vi "Error Cluster to Array.vi"(10 "error in (no error)":errorcluster) -> (2 "Error Array":string[](array[string]))   [LabVIEW 2019, in "Logger.Error.lvlib" / "Logger.Error.lvclass"]
uses:
  Logger.Error.lvclass
  <vilib>/Utility/error.llb/DialogType.ctl
  <userlib>/_OpenG.lib/string/string.llb/Trim Whitespace (String)__ogtk.vi
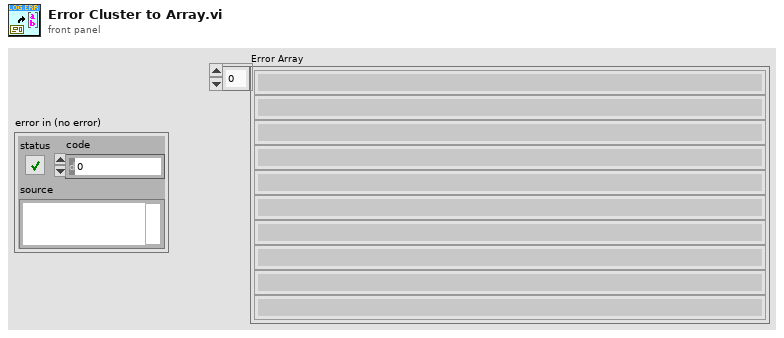
[diagram p1: front panel]
types:
  T1 = cluster{"Date":string, "Time":string, "Type":string, "Name":string, "Code":string, "Message":string, "Possible reason(s)":string, "Call Chain":string, "Calling Class":string}
  T2 = typedef "DialogType.ctl" = u16
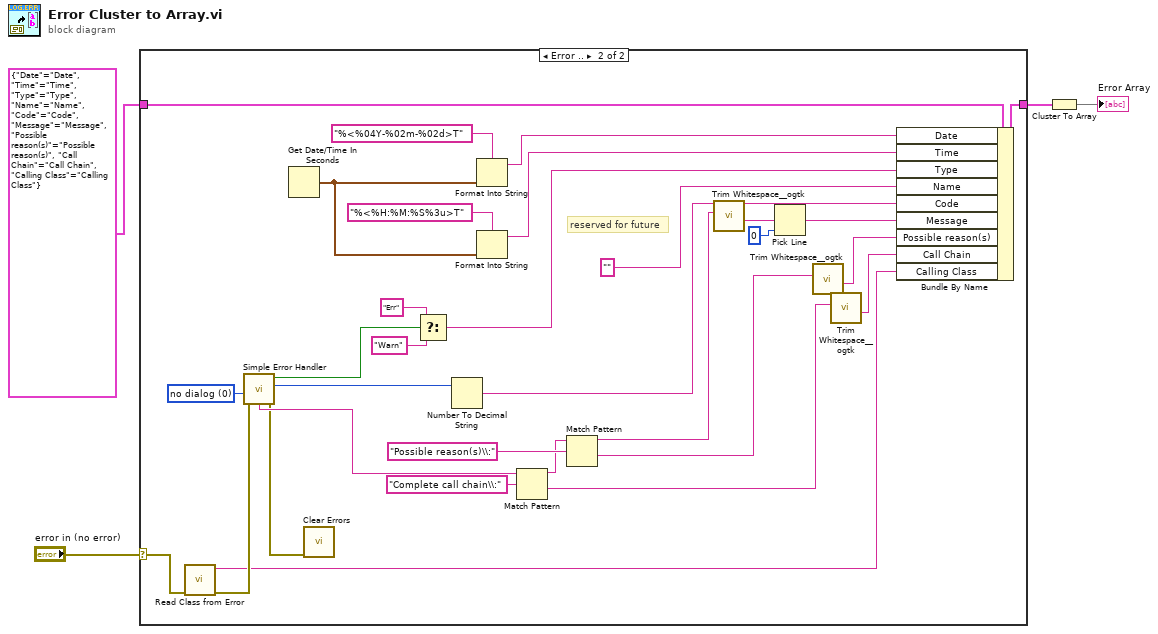
[diagram p0: block diagram]
diagram:
  n1 = case shown="Error .." "error in (no error)" {
    selector: "error in (no error)" -> [_ w12]
    tunnel: T1 {"Date"="Date", "Time"="Time", "Type"="Type", "Name"="Name", "Code"="Code", "Message"="Message", "Possible reason(s)"="Possible reason(s)", "Call Chain"="Call Chain", "Calling Class"="Calling Class"} ("Cluster") -> [w5 w31]
    tunnel: [w5 w32] -> w2
    frame No Error {
    }
    frame Error {
      w36 = T2 0 items=["no dialog", "OK message", "continue or stop message", "OK message + warnings", "continue/stop + warnings"] ("type of dialog (OK msg:1)")
      # "reserved for future"
      n2 = call "Read Class from Error.vi"("Error in"=w12) -> ("Error out"=w11:errorcluster, "Class"=w10:string)  [unwired: 8 in, 1 out]
      n3 = call <vilib>:"Simple Error Handler.vi"("type of dialog (OK msg:1)"=w36, "error in (no error)"=w11) -> ("error?"=w35:bool, "code out"=w25:i32, "error out"=w9:errorcluster, "message"=w13:string)  [unwired: 3 in, 1 out]
      n4 = Get Date/Time In Seconds() -> (seconds since 1Jan1904=w23:timestamp)
      n5 = call <vilib>:"Clear Errors.vi"("error in (no error)"=w9) -> ()  [unwired: 5 in, 2 out]
      n6 = Select(t="Err", s=w35, f="Warn") -> (s? t:f=w26:string)
      n7 = Number To Decimal String(number=w25) -> (decimal integer string=w24:string)  [unwired: 1 out]
      n8 = Format Into String(format string="%<%04Y-%02m-%02d>T", w23) -> (resulting string=w28:string)  [unwired: 2 in, 1 out]
      n9 = Format Into String(format string="%<%H:%M:%S%3u>T", w23) -> (resulting string=w27:string)  [unwired: 2 in, 1 out]
      n10 = Match Pattern(string=w13, regular expression="Complete call chain\\:") -> (before substring=w19:string, after substring=w18:string)  [unwired: 1 in, 2 out]
      n11 = Match Pattern(string=w19, regular expression="Possible reason(s)\\:") -> (before substring=w16:string, after substring=w17:string)  [unwired: 1 in, 2 out]
      n12 = call-poly <userlib>:"Trim Whitespace__ogtk.vi"("String in"=w16) -> ("String out"=w7:string)  [unwired: 6 in]
      n13 = Pick Line(multi-line string=w7, line index=0) -> (output string=w8:string)  [unwired: 1 in]
      n14 = call-poly <userlib>:"Trim Whitespace__ogtk.vi"("String in"=w17) -> ("String out"=w15:string)  [unwired: 6 in]
      n15 = call-poly <userlib>:"Trim Whitespace__ogtk.vi"("String in"=w18) -> ("String out"=w14:string)  [unwired: 6 in]
      n16 = Bundle By Name(cluster=w31, "Date"=w28, "Time"=w27, "Type"=w26, "Name"="", "Code"=w24, "Message"=w8, "Possible reason(s)"=w15, "Call Chain"=w14, "Calling Class"=w10) -> (w32:T1)
    }
  }
  n17 = Cluster To Array(cluster=w2) -> (array=→"Error Array":string[])
